vi "Ramp Gen.vi"() -> ()   [LabVIEW 2012]
uses:
  <vilib>/Analysis/1siggen.llb/Ramp Pattern by Samples.vi
  <vilib>/Analysis/NI_AALBase.lvlib
panel:
  out "Numeric 2":dbl
  out "Numeric":dbl
  in  "Scan Size":i32
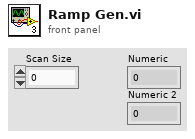
[diagram p1: front panel]
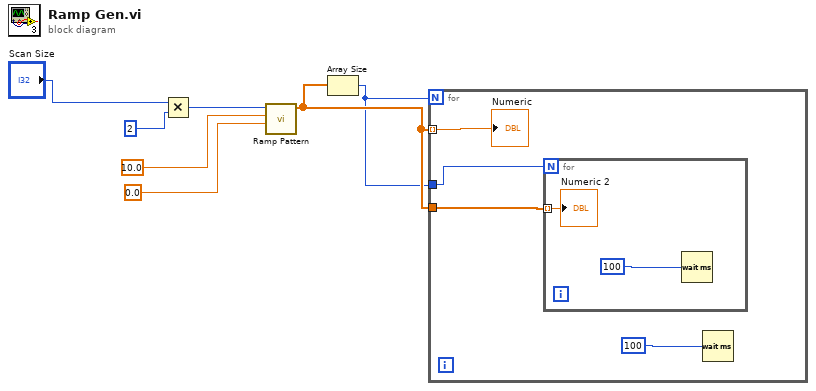
[diagram p0: block diagram]
diagram:
  n1 = Multiply(x="Scan Size", y=2) -> (x*y=w5:i32)
  n2 = call-poly <vilib>:"Ramp Pattern.vi"("start"=0.0, "end"=10.0, "samples"=w5) -> ("Ramp Pattern"=w2:dbl[])  [unwired: 7 in, 1 out]
  n3 = Array Size(array=w2) -> (size(s)=w1:i32)
  n4 = for {
    N: w1 -> [_]
    tunnel: w2 -> [w11] mode=indexing
    tunnel: w2 -> [w9]
    tunnel: w1 -> [w8]
    n5 = for {
      N: w8 -> [_]
      tunnel: w9 -> [w13] mode=indexing
      n6 = Wait (ms)(milliseconds to wait=u32 100) -> ()  [unwired: 1 out]
      "Numeric 2" <- w13
    }
    n7 = Wait (ms)(milliseconds to wait=u32 100) -> ()  [unwired: 1 out]
    "Numeric" <- w11
  }
